vi "Report Core.vi"(8 "error in":errorcluster, 9 "Received":path, 10 "Approved":path, 11 "Report With WinMerge in":refnum<class "Report With WinMerge.lvclass">) -> (0 "error out":errorcluster, 2 "Worked?":bool, 3 "Report With WinMerge out":refnum<class "Report With WinMerge.lvclass">)   [LabVIEW 2020, in "Approval Tests.lvlib" / "Report With WinMerge.lvclass"]
uses:
  Report With WinMerge.lvclass
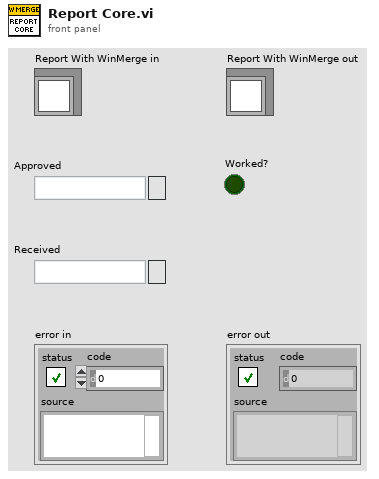
[diagram p1: front panel]
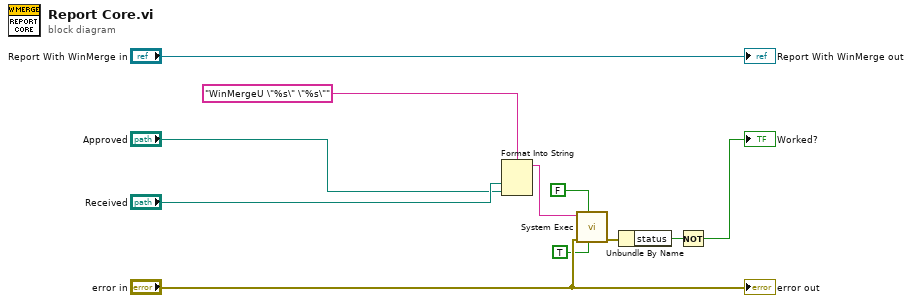
[diagram p0: block diagram]
diagram:
  n1 = Format Into String(format string="WinMergeU \"%s\" \"%s\"", "Received", "Approved") -> (resulting string=w7:string)  [unwired: 2 in, 1 out]
  n2 = call <vilib>:"System Exec.vi"("run minimized? (F)"=TRUE, "wait until completion? (T)"=FALSE, "error in (no error)"="error in", "command line"=w7) -> ("error out"=w11:errorcluster)  [unwired: 4 in, 3 out]
  n3 = Unbundle By Name(w11) -> ("status"=w3:bool)
  n4 = Not(x=w3) -> (.not. x?=→"Worked?":bool)
  "error out" <- "error in"
  "Report With WinMerge out" <- "Report With WinMerge in"
